vi "Sandbox Calc A P0.vi"() -> ()   [LabVIEW 2019]
uses:
  <vilib>/addons/_JKI.lib/FPGA_Basic_Components/Counter_32bit JKI_FPGA.vi
  <vilib>/Analysis/NI_AALPro.lvlib
  <vilib>/addons/_JKI.lib/FPGA_Basic_Components/JKI_BasicFPGA_Functions JKI_FPGA.lvlib
panel:
  out "Counter Out":u32
  in  "U pump 2":dbl[](array[numeric])=[10.0, 9.0, 8.0, 7.0, 6.0, 5.0, 4.0, 3.0, 2.0, 1.0, 0.0]
  in  "P pump 2":dbl[](array[numeric])=[5.06, 5.05, 5.05, 5.05, 4.68, 4.03, 3.32, 2.4, 1.87, 1.24, 0.54]
  in  "U haskel":dbl[](array[numeric])=[0.3, 0.4, 0.5, 0.6, 0.7]
  in  "P haskel":dbl[](array[numeric])=[11.93, 19.09, 25.85, 32.9, 40.07]
  in  "index":i32
  out "XY Graph":cluster{"U":dbl[], "P":dbl[]}[](graph)
  out "residue":dbl
  out "P0":dbl
  out "A":dbl
  in  "U pump":dbl[](array[numeric])=[1.0, 2.0, 3.0, 4.0, 5.0, 6.0, 6.0, 5.0, 4.0, 3.0, 2.0, 1.0]
  in  "P pump":dbl[](array[numeric])=[0.89, 1.57, 2.41, 3.18, 3.91, 4.57, 4.66, 4.02, 3.32, 2.44, 1.89, 1.32]
  # "P = A * U + P0"
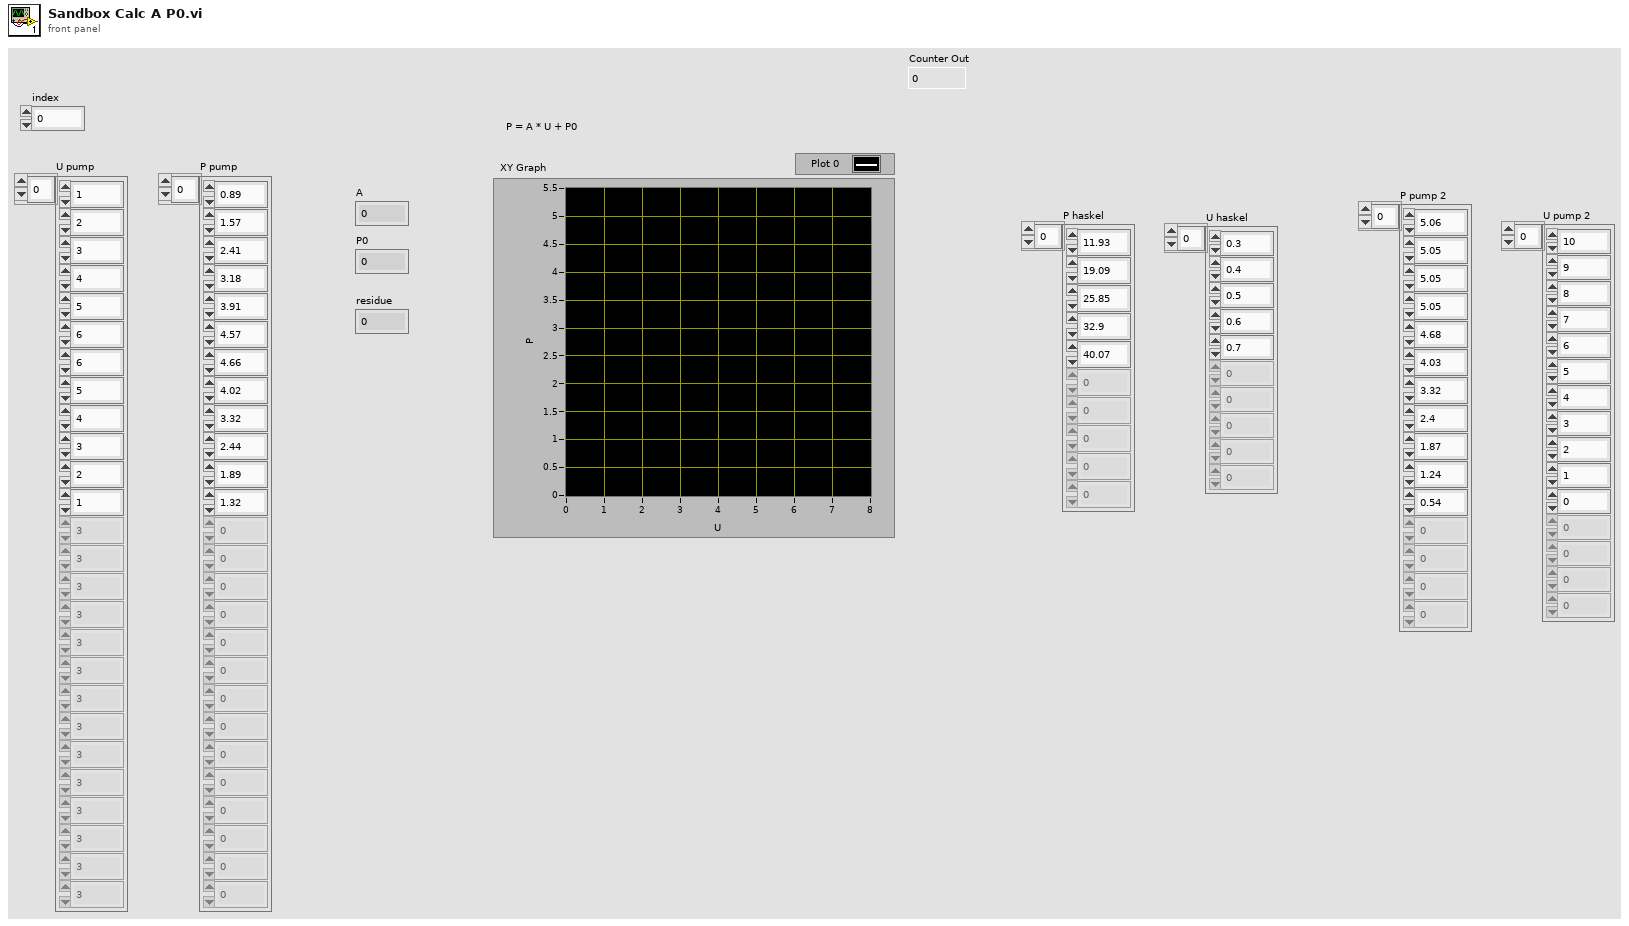
[diagram p1: front panel]
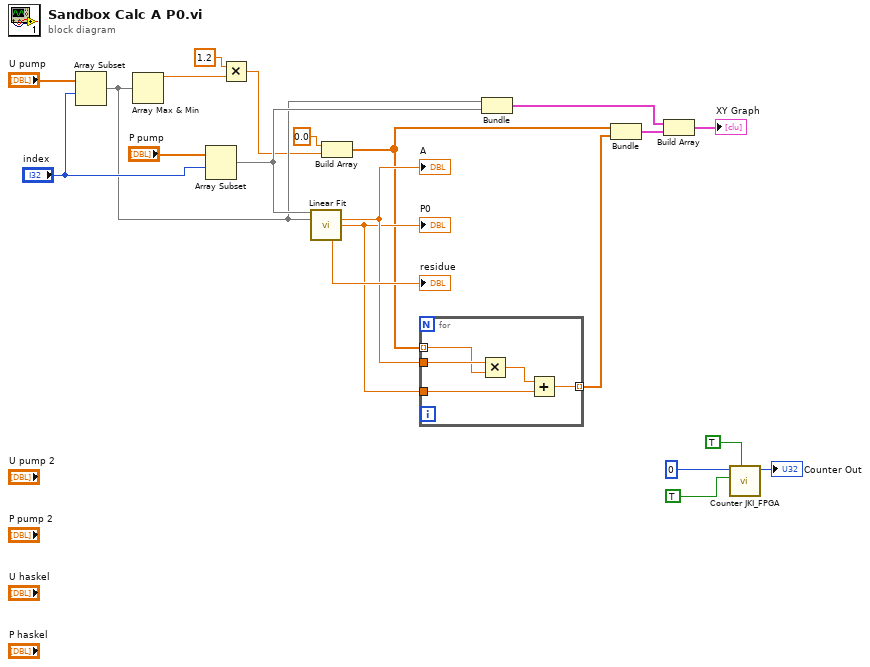
[diagram p0: block diagram]
diagram:
  n1 = Array Subset(array="U pump", index="index") -> (w8:dbl[])  [unwired: 1 in]
  n2 = Array Max & Min(array=w8) -> (max value=w7:dbl)  [unwired: 3 out]
  n3 = Array Subset(array="P pump", index="index") -> (w12:dbl[])  [unwired: 1 in]
  n4 = Multiply(x=1.2, y=w7) -> (x*y=w5:dbl)
  n5 = call <vilib>:"Linear Fit.vi"("Y"=w12, "X"=w8) -> ("slope"=w19:dbl, "intercept"=w18:dbl, "residue"=→"residue":dbl)  [unwired: 9 in, 2 out]
  "A" <- w19
  "P0" <- w18
  n6 = Build Array(0.0 ("element"), w5) -> (w9:dbl[])
  n7 = for {
    tunnel: w9 -> [w25] mode=indexing
    tunnel: w19 -> [w26]
    tunnel: w18 -> [w23]
    tunnel: [w22] -> w17 mode=indexing
    n8 = Multiply(x=w26, y=w25) -> (x*y=w24:dbl)
    n9 = Add(x=w24, y=w23) -> (x+y=w22:dbl)
  }
  n10 = Bundle(w8, w12) -> (w20:cluster{dbl[], dbl[]})  [unwired: 1 in]
  n11 = Bundle(w9, w17) -> (w15:cluster{dbl[], dbl[]})  [unwired: 1 in]
  n12 = Build Array(w20, w15) -> (→"XY Graph":cluster{dbl[], dbl[]}[])
  n13 = call-poly <vilib>:"Counter JKI_FPGA.vi"("Reset? (F)"=TRUE, "Count Up? (T)"=TRUE, "Initial Value in"=u32 0) -> ("Counter Out"=→"Counter Out":u32)  [unwired: 8 in]
